vi "Get_Day_File_Client.vi"(4 "Use Full Res Files":bool, 5 "Averaging Time (min)":dbl=5.0, 6 "End time":timestamp, 7 "Start time":timestamp, 8 "Channel Names":string[](array[string]), 9 "Data folder location":path=path "/G4-2-HD/Enflo Data/Server Day Files") -> (0 "Files with wrong times":path[](array[path]), 1 "All Channel Names":string[](array[string]), 2 "Data":dbl[][](array[numeric]), 3 "Times":dbl[](array[numeric]))   [LabVIEW 2022 SP3]
panel:
  out "stringData":string[][](array[string])
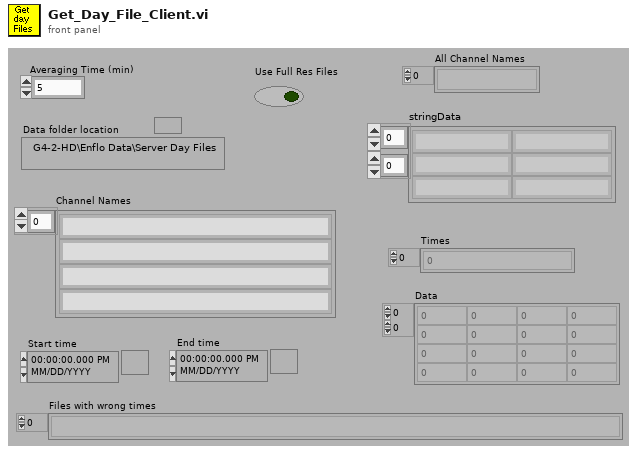
[diagram p1: front panel]
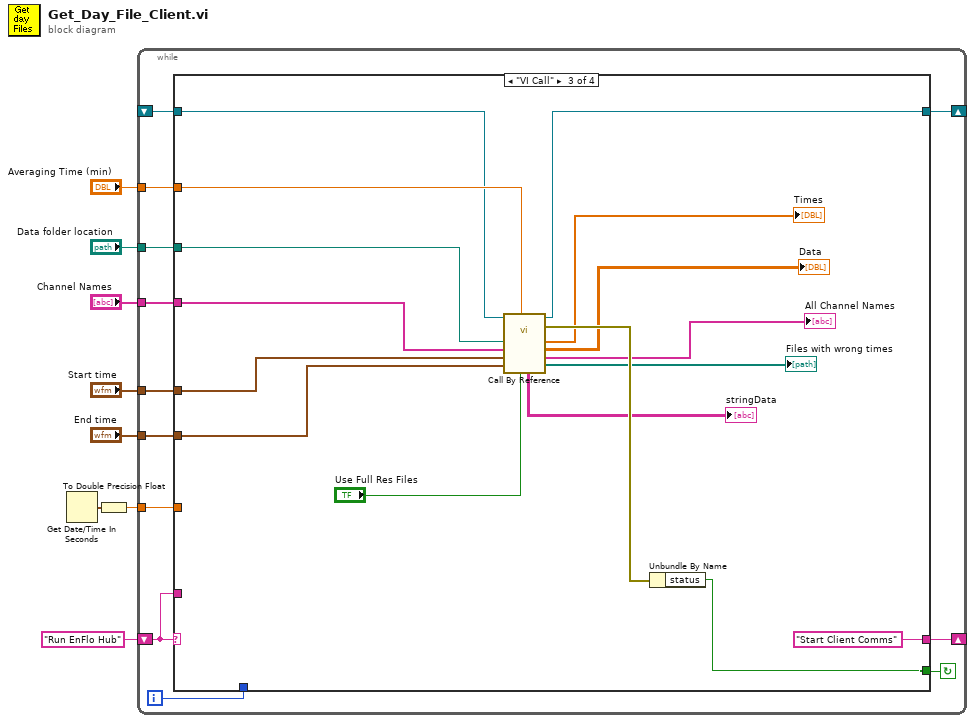
[diagram p0: block diagram]
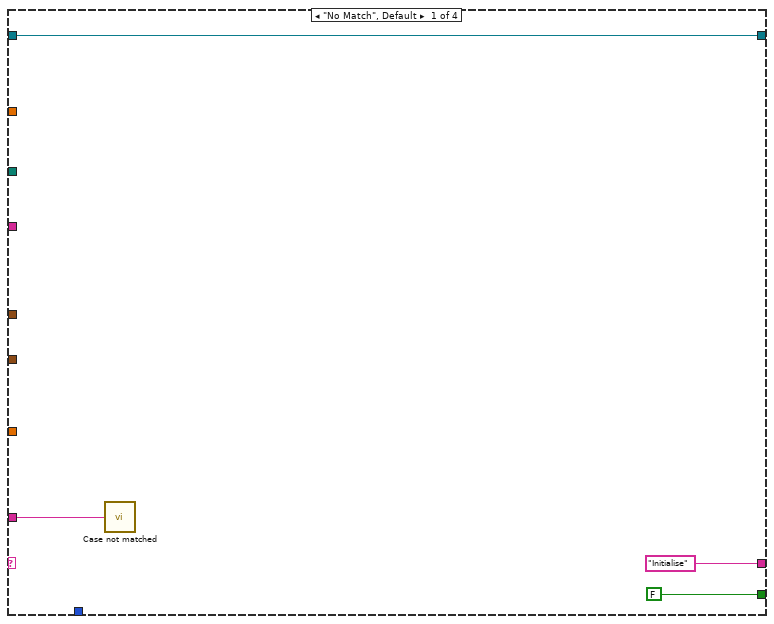
[diagram p2: hidden frame]
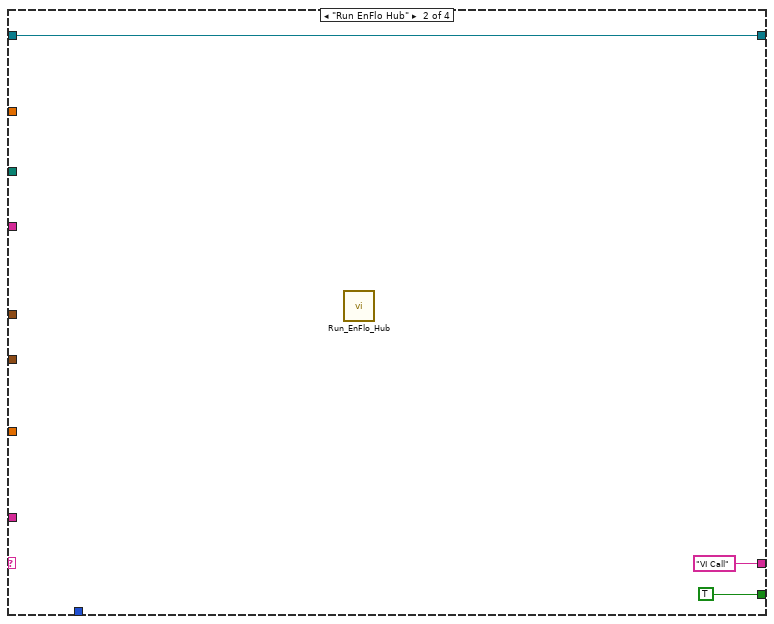
[diagram p3: hidden frame]
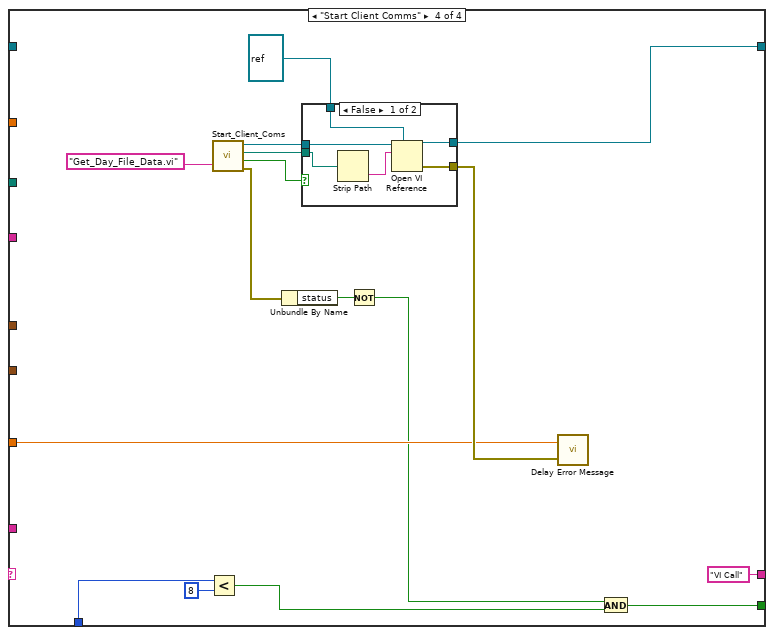
[diagram p4: hidden frame]
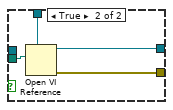
[diagram p5: hidden frame]
diagram:
  n1 = Get Date/Time In Seconds() -> (seconds since 1Jan1904=w2:timestamp)
  n2 = To Double Precision Float(number=w2) -> (double precision float=w1:dbl)
  n3 = while {
    shift-left: "Run EnFlo Hub" -> [w18]
    shift-right: [w19] -> _
    shift-right: [w12] -> _
    shift-left: _ -> [w11]
    tunnel: "Data folder location" -> [w17]
    tunnel: "Channel Names" -> [w16]
    tunnel: "Start time" -> [w15]
    tunnel: "End time" -> [w14]
    tunnel: "Averaging Time (min)" -> [w13]
    tunnel: w1 -> [w9]
    i -> [w10]
    stop <- w20 continue-if-true
    n4 = case shown="\"VI Call\"" w18 {
      tunnel: [FALSE TRUE w36 w44] -> w20
      tunnel: ["Initialise" "VI Call" "Start Client Comms" "VI Call"] -> w19
      tunnel: w18 -> [w21 _ _ _]
      tunnel: w17 -> [_ _ w42 _]
      tunnel: w16 -> [_ _ w41 _]
      tunnel: w15 -> [_ _ w40 _]
      tunnel: w14 -> [_ _ w39 _]
      tunnel: w13 -> [_ _ w38 _]
      tunnel: [w22 w26 w30 w54] -> w12
      tunnel: w11 -> [w22 w26 w31 _]
      tunnel: w10 -> [_ _ _ w52]
      tunnel: w9 -> [_ _ _ w49]
      frame "No Match", Default {
        n5 = call "Case not matched.vi"("Case Name not Matched"=w21) -> ()
      }
      frame "Run EnFlo Hub" {
        n6 = call "Run_EnFlo_Hub.vi"() -> ()  [unwired: 1 in, 7 out]
      }
      frame "VI Call" {
        n7 = call-by-ref "?"(reference=w31, "Use Full Res Files"="Use Full Res Files", "Averaging Time (min)"=w38, "End time"=w39, "Start time"=w40, "Channel Names"=w41, "Data folder location"=w42) -> (reference out=w30:refnum<vi>, error out=w37:errorcluster, "Files with wrong times"=→"Files with wrong times":path[], "All Channel Names"=→"All Channel Names":string[], "Data"=→"Data":dbl[][], "Times"=→"Times":dbl[], "stringData"=→"stringData":string[][])  [unwired: 2 in]
        n8 = Unbundle By Name(w37) -> ("status"=w36:bool)
      }
      frame "Start Client Comms" {
        n9 = Less?(x=w52, y=8) -> (x < y?=w46:bool)
        n10 = call "Start_Client_Coms.vi"("VI name to run on server"="Get_Day_File_Data.vi") -> ("LabVIEW application reference"=w57:refnum<vi>, "Checked VI name"=w59:path, "Local Call"=w58:bool, "Error cluster"=w47:errorcluster)  [unwired: 1 in]
        n11 = Unbundle By Name(w47) -> ("status"=w48:bool)
        n12 = case shown="False" w58 {
          tunnel: refnum<vi> refnum ("trivial.vi type") -> [w61 w69]
          tunnel: w59 -> [w62 w68]
          tunnel: w57 -> [w60 _]
          tunnel: [w64 w67] -> w50
          tunnel: [w63 w66] -> w54
          frame False {
            n13 = Strip Path(path=w62) -> (name=w65:string)  [unwired: 1 out]
            n14 = Open VI Reference(type specifier VI Refnum (for type only)=w61, application reference (local)=w60, vi path=w65) -> (vi reference=w63:refnum<vi>, error out=w64:errorcluster)  [unwired: 1 in, 2 out]
          }
          frame True {
            n15 = Open VI Reference(type specifier VI Refnum (for type only)=w69, vi path=w68) -> (vi reference=w66:refnum<vi>, error out=w67:errorcluster)  [unwired: 1 in, 3 out]
          }
        }
        n16 = Not(x=w48) -> (.not. x?=w45:bool)
        n17 = call "Delay Error Message.vi"("error in (no error)"=w50, "Seconds since 1904"=w49) -> ()  [unwired: 2 in]
        n18 = And(x=w45, y=w46) -> (x .and. y?=w44:bool)
      }
    }
  }
